vi "GetInstanceDefault.vi"(8 "error in (no error)":errorcluster, 11 "Subsystem in":refnum<class "SubsystemData.lvclass">) -> (0 "error out":errorcluster, 1 "Instance Default":refnum<class "SubsystemData.lvclass">, 3 "Subsystem out":refnum<class "SubsystemData.lvclass">)   [LabVIEW 2017, in "SubsystemData.lvclass"]
uses:
  SubsystemData/SubsystemData.lvclass
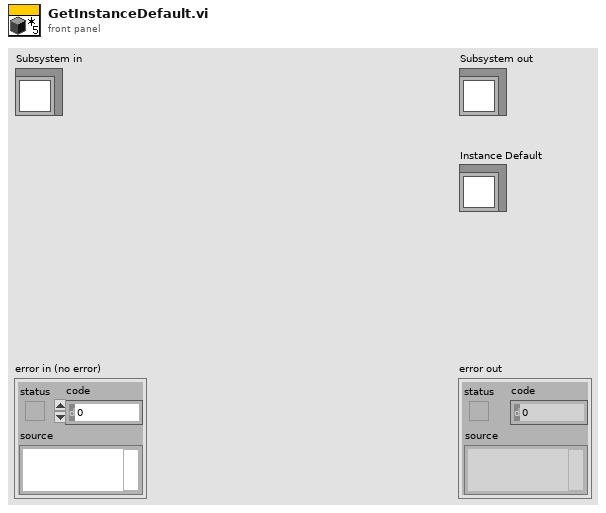
[diagram p1: front panel]
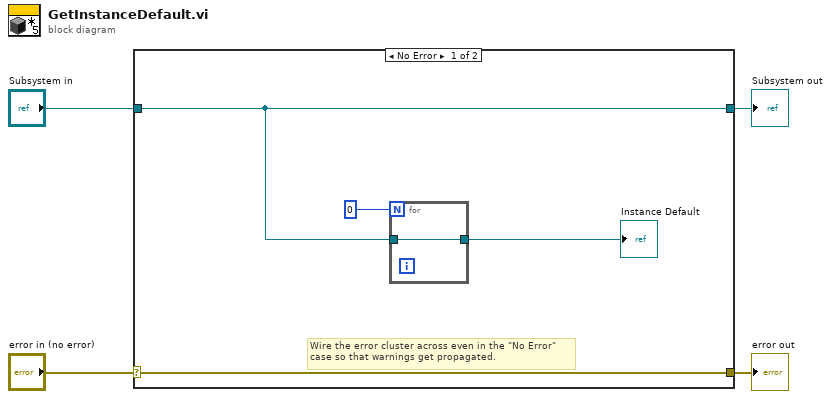
[diagram p0: block diagram]
diagram:
  n1 = case shown="No Error" "error in (no error)" {
    selector: "error in (no error)" -> [w8 w11]
    tunnel: [w8 w11] -> w3
    tunnel: [w6 w10] -> w1
    tunnel: "Subsystem in" -> [w6 w10]
    frame No Error {
      # "Wire the error cluster across even in the \"No Error\"\ncase so that warnings get propagated."
      n2 = for {
        N: 0 -> [_]
        tunnel: [w9] -> w5
        tunnel: w6 -> [w9]
      }
      "Instance Default" <- w5
    }
    frame Error {
    }
  }
  "error out" <- w3
  "Subsystem out" <- w1
